vi "Write 7z config.vi"(8 "error in (no error)":errorcluster, 11 "PostBuildSupport in":refnum<class "PostBuildSupport.lvclass">) -> (0 "error out":errorcluster, 3 "PostBuildSupport out":refnum<class "PostBuildSupport.lvclass">)   [LabVIEW 2016, in "PostBuildSupport.lvclass"]
uses:
  PostBuildSupport.lvclass
  PostBuildSupport.lvclass/PostBuildSupport.ctl
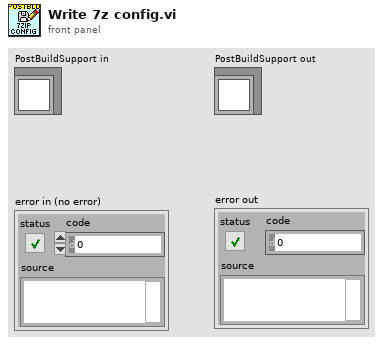
[diagram p1: front panel]
types:
  T1 = enum16{"open", "replace", "create", "open or create", "replace or create", "replace or create with confirmation"}
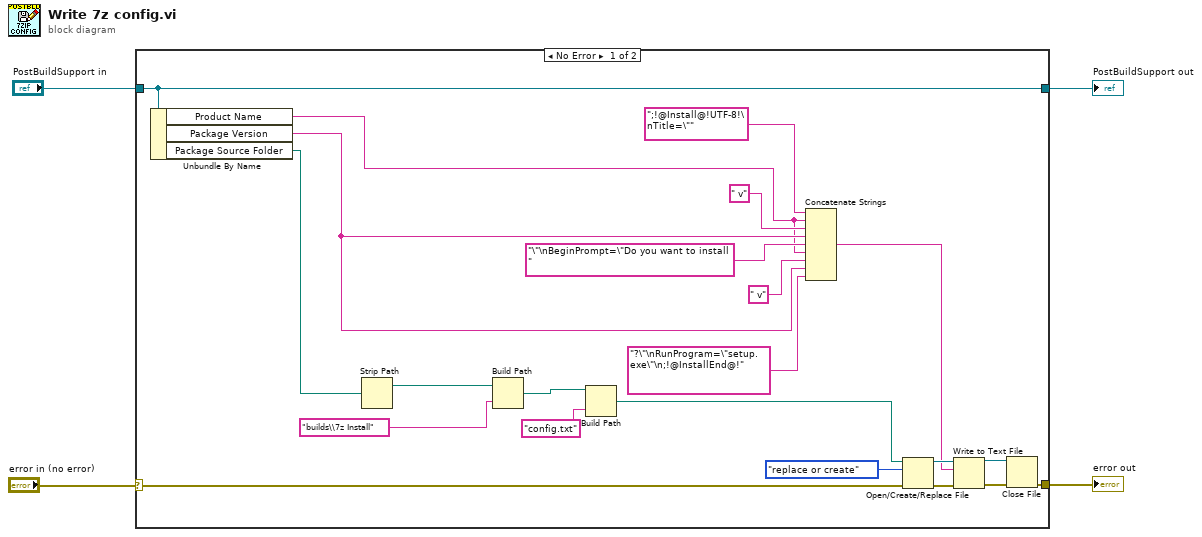
[diagram p0: block diagram]
diagram:
  n1 = case shown="No Error" "error in (no error)" {
    selector: "error in (no error)" -> [w6 w27]
    tunnel: [w16 w27] -> w4
    tunnel: "PostBuildSupport in" -> [w7 w28]
    tunnel: [w7 w28] -> w2
    frame No Error {
      n2 = Unbundle By Name(w7) -> ("Product Name"=w5:string, "Package Version"=w8:string, "Package Source Folder"=w9:path)
      n3 = Strip Path(path=w9) -> (stripped path=w25:path)  [unwired: 1 out]
      n4 = Build Path(base path=w25, name or relative path="builds\\7z Install") -> (appended path=w15:path)
      n5 = Build Path(base path=w15, name or relative path="config.txt") -> (appended path=w20:path)
      n6 = Concatenate Strings(";!@Install@!UTF-8!\nTitle=\"" ("Name of target (My Computer)"), w5, " v" ("Name of target (My Computer)"), w8, "\"\nBeginPrompt=\"Do you want to install " ("Name of target (My Computer)"), w5, " v" ("Name of target (My Computer)"), w8, "?\"\nRunProgram=\"setup.exe\"\n;!@InstallEnd@!" ("Name of target (My Computer)")) -> (w22:string)
      n7 = Open/Create/Replace File(file path (use dialog)=w20, error in=w6, operation (0:open)=T1."replace or create") -> (refnum out=w23:refnum<file>, error out=w21:errorcluster)  [unwired: 3 in, 1 out]
      n8 = Write to Text File(file (use dialog)=w23, text=w22, error in=w21) -> (refnum out=w17:refnum<file>, error out=w18:errorcluster)  [unwired: 1 in, 1 out]
      n9 = Close File(refnum=w17, error in=w18) -> (error out=w16:errorcluster)  [unwired: 1 out]
    }
    frame Error {
    }
  }
  "error out" <- w4
  "PostBuildSupport out" <- w2
